vi "configureTriggering.vi"(8 "error in (no error)":errorcluster, 11 "AndorIKonAcquisitor in":refnum<class "AndorIKonAcquisitor.lvclass">) -> (0 "error out":errorcluster, 3 "AndorIKonAcquisitor out":refnum<class "AndorIKonAcquisitor.lvclass">)   [LabVIEW 2011, in "Hardware.lvlib" / "Channels.lvlib" / "AndorIKonAcquisitor.lvclass"]
uses:
  AndorIKonAcquisitor.lvclass
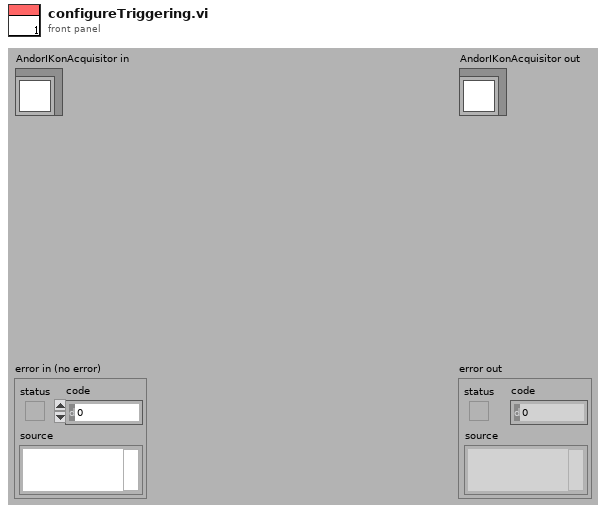
[diagram p1: front panel]
types:
  T1 = cluster{"Trigger Mode":dbl, "Fast Triggering":bool}
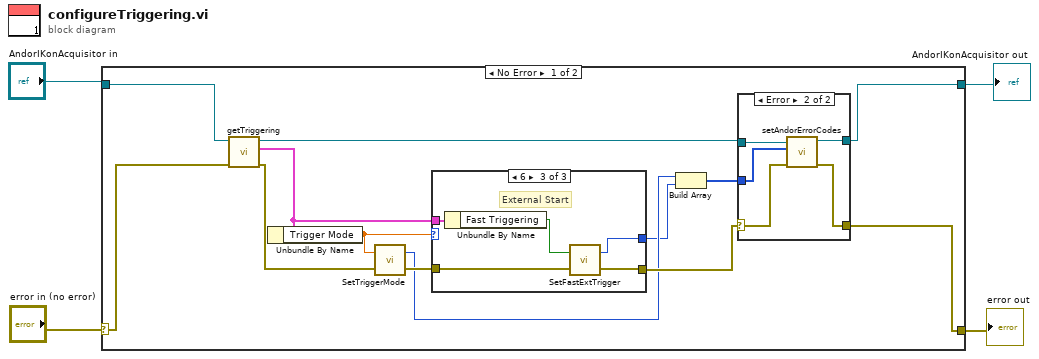
[diagram p0: block diagram]
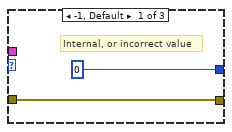
[diagram p3: hidden frame]
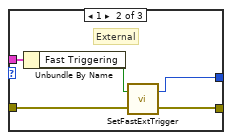
[diagram p4: hidden frame]
diagram:
  n1 = case shown="No Error" "error in (no error)" {
    selector: "error in (no error)" -> [w15 w37]
    tunnel: "AndorIKonAcquisitor in" -> [w16 w38]
    tunnel: [w5 w38] -> w1
    tunnel: [w8 w37] -> w2
    frame No Error {
      n2 = call-dynamic "getTriggering.vi"("error in (no error)"=w15, "CameraAcquisitor.lvclass in"=w16) -> ("error out"=w14:errorcluster, "Triggering"=w12:T1, "CameraAcquisitor.lvclass out"=w11:refnum<class "AndorIKonAcquisitor.lvclass">)  [unwired: 7 in]
      n3 = Unbundle By Name(w12) -> ("Trigger Mode"=w13:dbl)
      n4 = call <userlib>:"SetTriggerMode.vi"("error in (no error)"=w14, "mode"=w13) -> ("error out"=w17:errorcluster, "DLL error code"=w7:u32)
      n5 = case shown="6" w13 {
        tunnel: w17 -> [w26 w31 w36]
        tunnel: [w26 w30 w35] -> w9
        tunnel: [0 w29 w34] -> w6
        tunnel: w12 -> [_ w28 w33]
        frame -1, Default {
          # "Internal, or incorrect value"
        }
        frame 1 {
          # "External"
          n6 = Unbundle By Name(w28) -> ("Fast Triggering"=w27:bool)
          n7 = call <userlib>:"SetFastExtTrigger.vi"("error in (no error)"=w31, "mode"=w27) -> ("error out"=w30:errorcluster, "DLL error code"=w29:u32)
        }
        frame 6 {
          # "External Start"
          n8 = Unbundle By Name(w33) -> ("Fast Triggering"=w32:bool)
          n9 = call <userlib>:"SetFastExtTrigger.vi"("error in (no error)"=w36, "mode"=w32) -> ("error out"=w35:errorcluster, "DLL error code"=w34:u32)
        }
      }
      n10 = Build Array(w7, w6) -> (w10:u32[])
      n11 = case shown="Error" w9 {
        selector: w9 -> [w19 w23]
        tunnel: w11 -> [w18 w24]
        tunnel: [w18 w21] -> w5
        tunnel: [w19 w22] -> w8
        tunnel: w10 -> [_ w20]
        frame No Error {
        }
        frame Error {
          n12 = call-dynamic "setAndorErrorCodes.vi"("error in (no error)"=w23, "Andor Error Codes"=w20, "AndorIKonAcquisitor.lvclass in"=w24) -> ("error out"=w22:errorcluster, "AndorIKonAcquisitor.lvclass out"=w21:refnum<class "AndorIKonAcquisitor.lvclass">)  [unwired: 7 in]
        }
      }
    }
    frame Error {
    }
  }
  "error out" <- w2
  "AndorIKonAcquisitor out" <- w1
